vi "SaveCreatePath.vi"(8 "error in":errorcluster, 9 "Exp Folder":string="<date>_exp<#>", 10 "ExperimentNumber":u32, 11 "BaseFolder":path) -> (0 "error out":errorcluster, 3 "appended path":path)   [LabVIEW 2016]
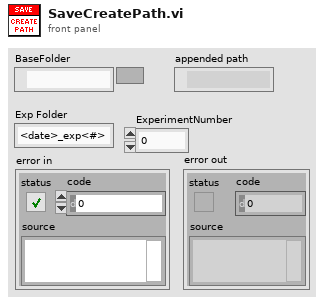
[diagram p1: front panel]
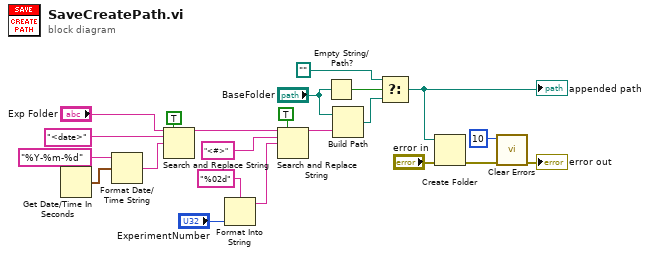
[diagram p0: block diagram]
diagram:
  n1 = Get Date/Time In Seconds() -> (seconds since 1Jan1904=w12:timestamp)
  n2 = Format Date/Time String(time format string (%c)="%Y-%m-%d", seconds (now)=w12) -> (date/time string=w9:string)  [unwired: 1 in]
  n3 = Search and Replace String(replace all?=TRUE ("replace all? (F)"), input string="Exp Folder", search string="<date>", replace string=w9) -> (result string=w16:string)  [unwired: 4 in, 3 out]
  n4 = Format Into String(format string="%02d", "ExperimentNumber") -> (resulting string=w13:string)  [unwired: 2 in, 1 out]
  n5 = Search and Replace String(replace all?=TRUE ("replace all? (F)"), input string=w16, search string="<#>", replace string=w13) -> (result string=w17:string)  [unwired: 4 in, 3 out]
  n6 = Empty String/Path?(string/path="BaseFolder") -> (empty?=w7:bool)
  n7 = Build Path(base path="BaseFolder", name or relative path=w17) -> (appended path=w5:path)
  n8 = Select(t=path "", s=w7, f=w5) -> (s? t:f=w4:path)
  "appended path" <- w4
  n9 = Create Folder(path (use dialog)=w4, error in="error in") -> (error out=w22:errorcluster)  [unwired: 1 in, 2 out]
  n10 = call <vilib>:"Clear Errors.vi"("error in (no error)"=w22, "specific error code to clear (0: all)"=10) -> ("error out"=→"error out":errorcluster)  [unwired: 4 in, 1 out]
